vi "19052 Get_test_STEPS_number.vi"(8 "error in (no error)":errorcluster, 11 "VISA resource in":refnum<visa-resource-name>) -> (0 "error out":errorcluster, 1 "# Active steps":u16 format="%.0p", 3 "VISA resource out":refnum<visa-resource-name>)   [LabVIEW 2015]
doc: "This VI retrieves the number of steps set in the instrument."
panel:
  out "output command":string
  # "Get # of active STEPs"
  # "This is valid for both: 19572 & 19052"
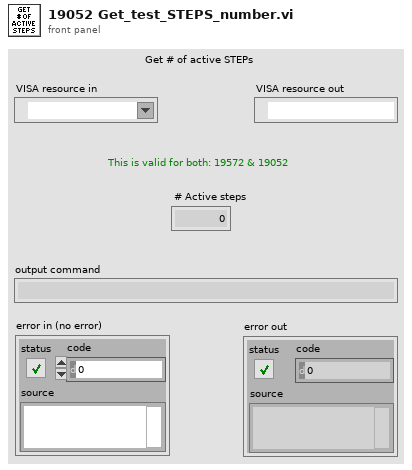
[diagram p1: front panel]
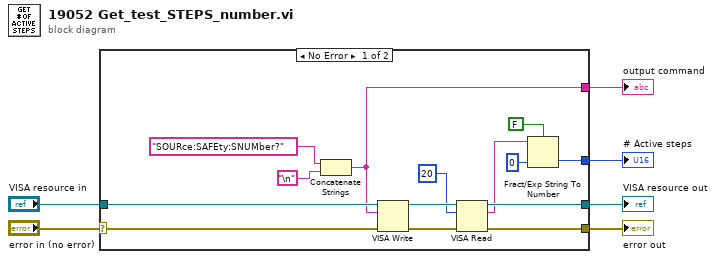
[diagram p0: block diagram]
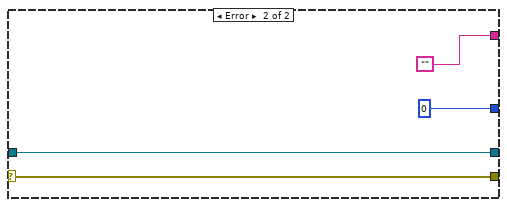
[diagram p2: hidden frame]
diagram:
  n1 = case shown="No Error" "error in (no error)" {
    selector: "error in (no error)" -> [w12 w23]
    tunnel: [w20 w23] -> w6
    tunnel: "VISA resource in" -> [w19 w24]
    tunnel: [w17 ""] -> w4
    tunnel: [w13 w24] -> w3
    tunnel: [w8 u16 0 ("offset past number")] -> w1
    frame No Error {
      n2 = Concatenate Strings("SOURce:SAFEty:SNUMber?", "\n") -> (w17:string)
      n3 = VISA Write(VISA resource name=w19, write buffer=w17, error in (no error)=w12) -> (VISA resource name out=w15:refnum<visa-resource-name>, error out=w16:errorcluster)  [unwired: 1 out]
      n4 = VISA Read(VISA resource name=w15, byte count=u32 20, error in (no error)=w16) -> (VISA resource name out=w13:refnum<visa-resource-name>, read buffer=w10:string, error out=w20:errorcluster)  [unwired: 1 out]
      n5 = Fract/Exp String To Number(use system decimal point (T)=FALSE, string=w10, default (0 dbl)=u16 0 ("default (0 DBL)")) -> (number=w8:u16)  [unwired: 1 in, 1 out]
    }
    frame Error {
    }
  }
  "error out" <- w6
  "VISA resource out" <- w3
  "output command" <- w4
  "# Active steps" <- w1
